vi "Module Cleanup.vi"(8 "error in (no error)":errorcluster, 11 "Telemetry Client in":refnum<class "Telemetry Client.lvclass">) -> (0 "error out":errorcluster, 3 "Telemetry Client out":refnum<class "Telemetry Client.lvclass">)   [LabVIEW 2020, in "VolatusTelemetry.lvlib" / "Telemetry Client.lvclass"]
uses:
  Telemetry Client.lvclass
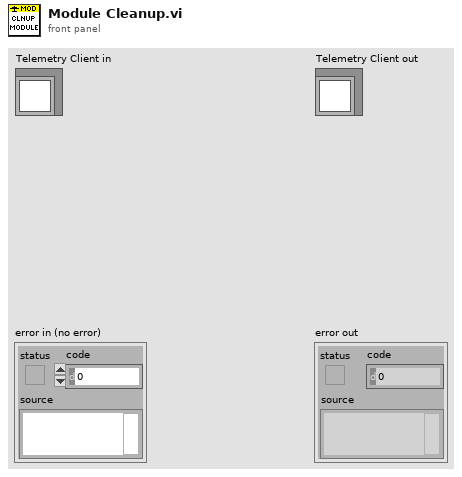
[diagram p1: front panel]
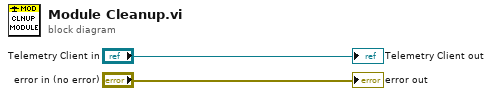
[diagram p0: block diagram]
diagram:
  "error out" <- "error in (no error)"
  "Telemetry Client out" <- "Telemetry Client in"
